vi "LoadRuleParserConfigurationPage.vi"(8 "error in (no error)":errorcluster, 9 "Selection":string, 11 "UIManager in":refnum<class "UIManager.lvclass">) -> (0 "error out":errorcluster, 1 "References":T1, 3 "UIManager out":refnum<class "UIManager.lvclass">)   [LabVIEW 2020, in "DependencyInspector.lvlib" / "UIManager.lvclass"]
uses:
  UIManager.lvclass
  Private/subReferenceData.ctl
  obj/Addons/ExtensionInterfaces.lvlibp/IConfigurationPage/Event_Stop.ctl
  obj/Addons/ExtensionInterfaces.lvlibp/IConfigurationPage/Event_Parameters.ctl
  UIManager.lvclass/UIManager.ctl
  DependencyInspector.lvlib
  obj/Addons/ExtensionInterfaces.lvlibp/IRuleFileParser/IRuleFileParser.lvclass
  obj/Addons/ExtensionInterfaces.lvlibp/IConfigurationPage/IConfigurationPage.lvclass
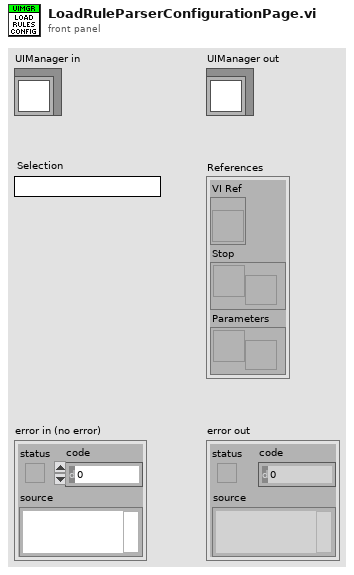
[diagram p1: front panel]
types:
  T1 = typedef "DependencyInspector.lvlib/subReferenceData.ctl" = cluster{"VI Ref":refnum<vi>, "Stop":refnum<user-event>, "Parameters":refnum<user-event>}
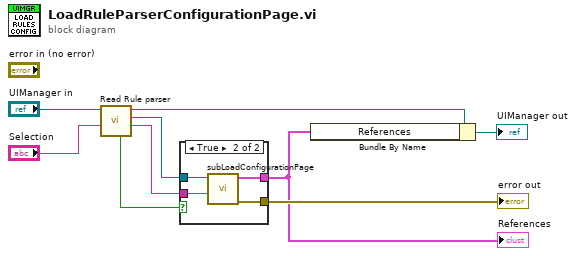
[diagram p0: block diagram]
diagram:
  n1 = call-dynamic "Read Rule parser.vi"("Selection"="Selection", "UIManager in"="UIManager in") -> ("Parameters"=w1:string, "IRuleFileParser.lvclass"=w3:refnum<class "IRuleFileParser.lvclass">, "UIManager out"=w2:refnum<class "UIManager.lvclass">, "found?"=w4:bool)  [unwired: 6 in]
  n2 = case shown="True" w4 {
    tunnel: w3 -> [_ w13]
    tunnel: [_ w12] -> w9
    tunnel: [_ w11] -> w8
    tunnel: w1 -> [_ w10]
    frame False {
    }
    frame True {
      n3 = call "subLoadConfigurationPage.vi"("Parameters"=w10, "Interface in"=w13) -> ("error out"=w12:errorcluster, "References"=w11:T1)  [unwired: 8 in]
    }
  }
  "error out" <- w9
  "References" <- w8
  n4 = Bundle By Name(cluster=w2, "References"=w8) -> (→"UIManager out":refnum<class "UIManager.lvclass">)
